vi "TestNewStructure.vi"() -> ()   [LabVIEW 2024]
uses:
  Library/Class/Renishaw-XL80_EMU/Renishaw-XL80_EMU.lvclass
panel:
  in  "Reset":bool
  out "Record":dbl
  out "GetLaserMeasurement 2":dbl
  out "Connect 2":bool
  in  "Boolean":bool
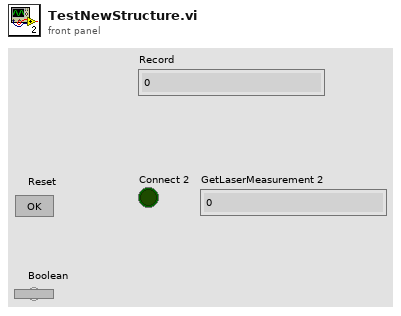
[diagram p1: front panel]
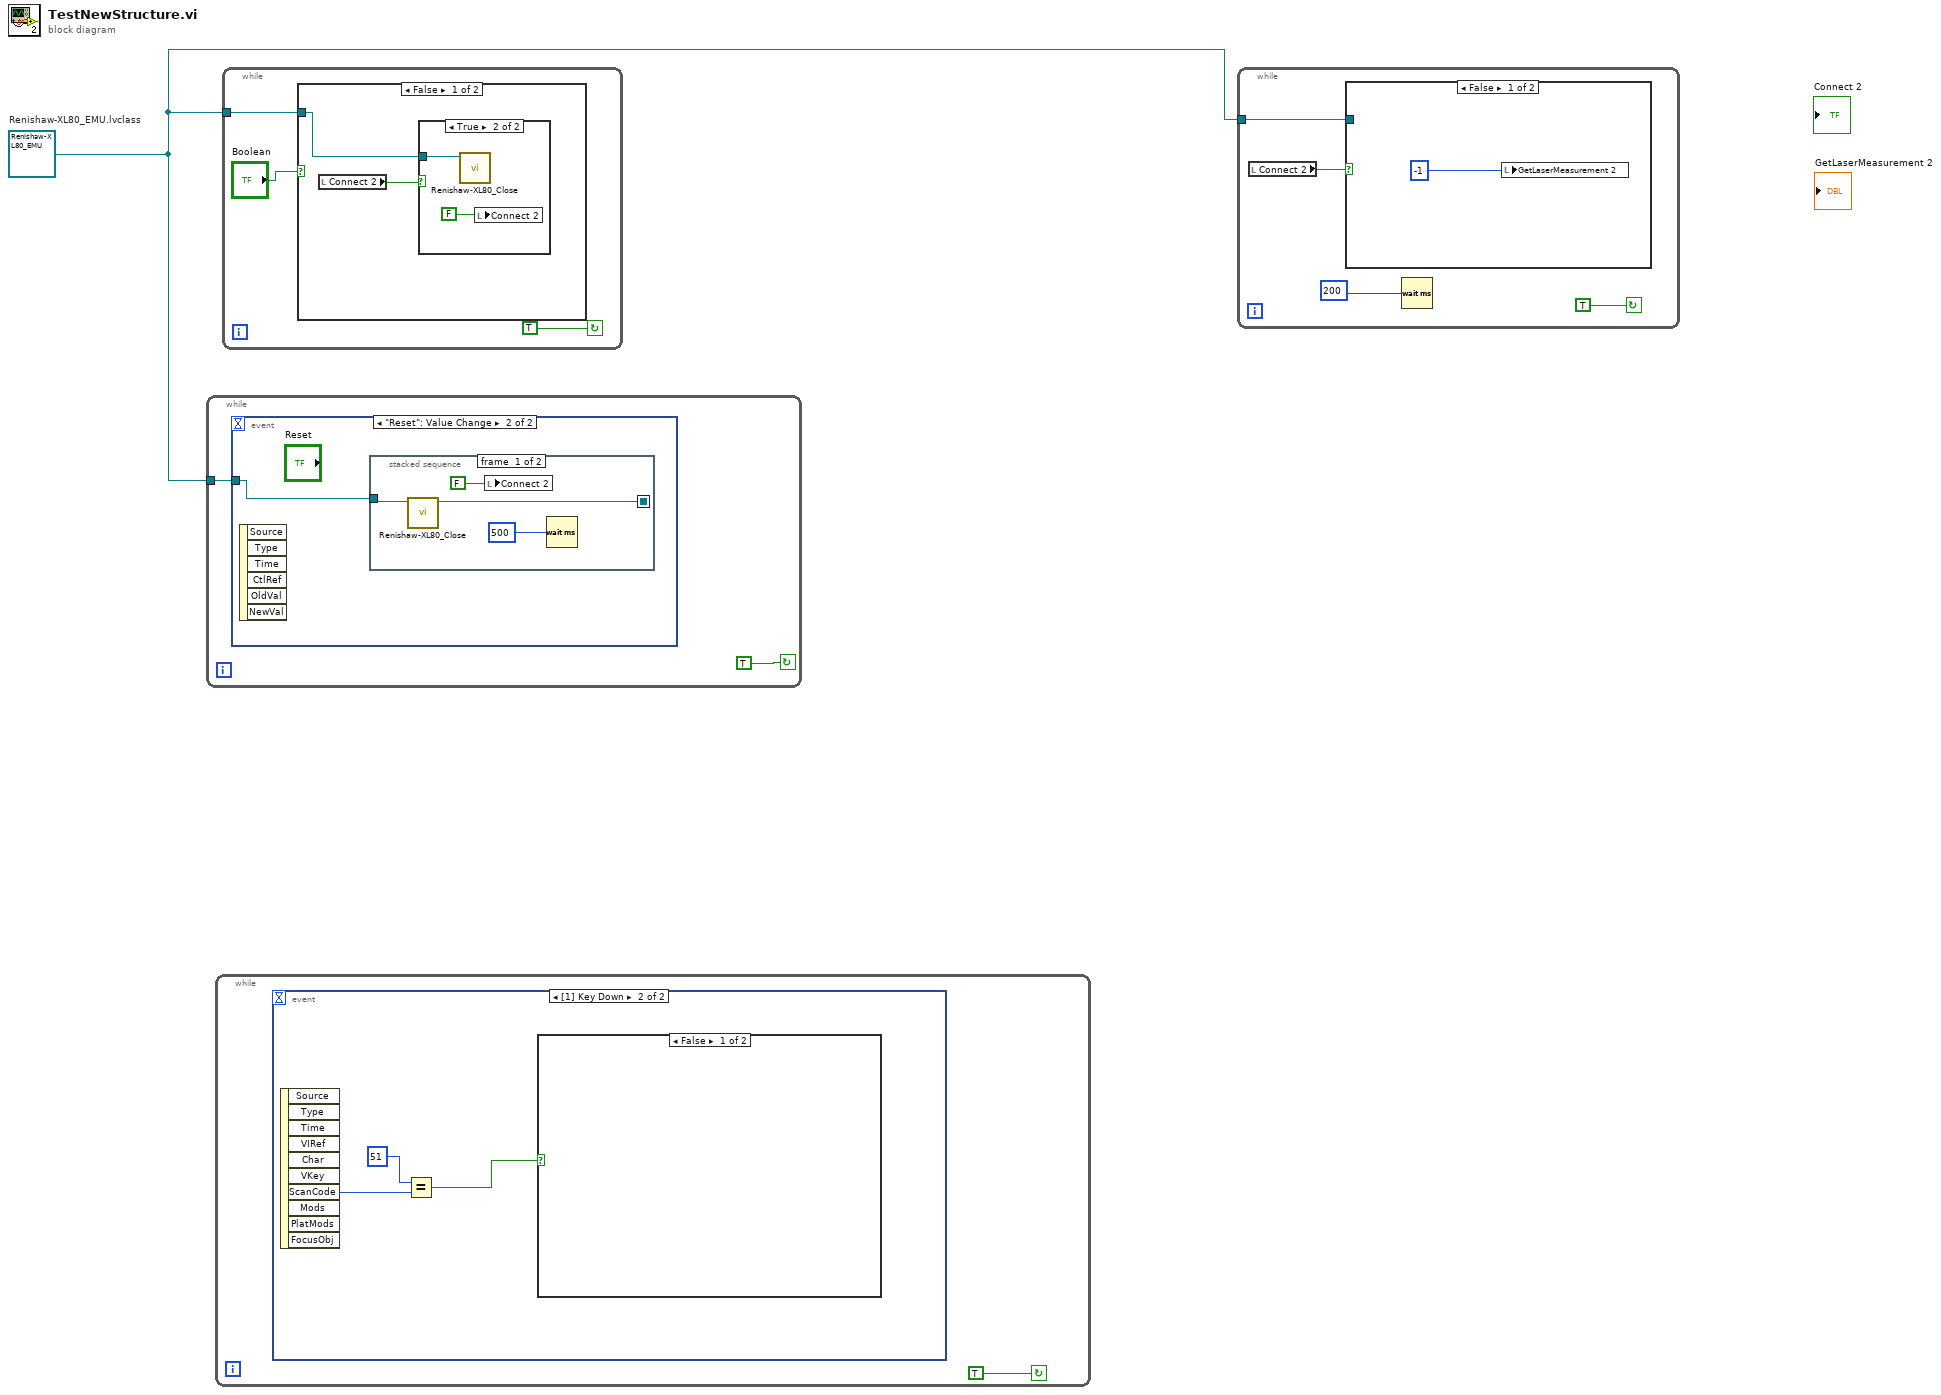
[diagram p0: block diagram]
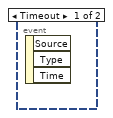
[diagram p2: hidden frame]
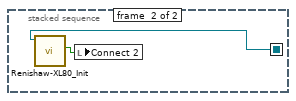
[diagram p3: hidden frame]
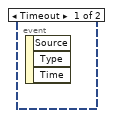
[diagram p4: hidden frame]
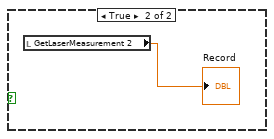
[diagram p5: hidden frame]
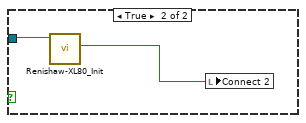
[diagram p7: hidden frame]
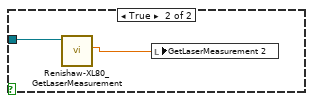
[diagram p8: hidden frame]
diagram:
  w1 = refnum<class "Renishaw-XL80_EMU.lvclass"> refnum  # Renishaw-XL80_EMU.lvclass
  n1 = while {
    tunnel: w1 -> [w3]
    stop <- TRUE continue-if-true
    n2 = event shown="[1] \"Reset\": Value Change" {
      selector: _ -> [_ _]
      dyn-events: _ -> [_ _]
      timeout: _ -> [_ _]
      tunnel: w3 -> [_ w4]
      event Timeout {
        n3 = event-data() -> ()  [unwired: 1 in, 3 out]
      }
      event "Reset": Value Change {
        n4 = event-data() -> ()  [unwired: 1 in, 6 out]
        n5 = stacked-sequence {
          seq-local: [w6 _] -> [_ w9]
          tunnel: w4 -> [w8 _]
          frame #0 {
            n6 = call-dynamic "Renishaw-XL80_Close.vi"("Renishaw-XL80_EMU in"=w8) -> ("Renishaw-XL80_EMU out"=w6:refnum<class "Renishaw-XL80_EMU.lvclass">)  [unwired: 9 in, 1 out]
            n7 = local write "Connect 2"(FALSE ("Connect 2")) -> ()
            n8 = Wait (ms)(milliseconds to wait=u32 500) -> ()  [unwired: 1 out]
          }
          frame #1 {
            n9 = call-dynamic "Renishaw-XL80_Init.vi"("Renishaw-XL80_EMU in"=w9) -> ("Connect"=w10:bool)  [unwired: 7 in, 3 out]
            n10 = local write "Connect 2"(w10) -> ()
          }
        }
      }
    }
  }
  n11 = while {
    stop <- TRUE continue-if-true
    n12 = event shown="[1] Key Down" {
      selector: _ -> [_ _]
      dyn-events: _ -> [_ _]
      timeout: _ -> [_ _]
      event Timeout {
        n13 = event-data() -> ()  [unwired: 1 in, 3 out]
      }
      event Key Down {
        n14 = event-data() -> ("ScanCode"=w13:i16)  [unwired: 1 in, 9 out]
        n15 = Equal?(x=i16 51 ("y"), y=w13) -> (x = y?=w12:bool)
        n16 = case shown="False" w12 {
          frame False {
          }
          frame True {
            n17 = local read "GetLaserMeasurement 2"() -> (→"Record":dbl)
          }
        }
      }
    }
  }
  n18 = while {
    tunnel: w1 -> [w17]
    stop <- TRUE continue-if-true
    n19 = case shown="False" "Boolean" {
      tunnel: w17 -> [w19 w23]
      frame False {
        n20 = local read "Connect 2"() -> (w20:bool)
        n21 = case shown="True" w20 {
          tunnel: w19 -> [_ w22]
          frame False {
          }
          frame True {
            n22 = call-dynamic "Renishaw-XL80_Close.vi"("Renishaw-XL80_EMU in"=w22) -> ()  [unwired: 9 in, 2 out]
            n23 = local write "Connect 2"(FALSE ("Connect")) -> ()
          }
        }
      }
      frame True {
        n24 = call-dynamic "Renishaw-XL80_Init.vi"("Renishaw-XL80_EMU in"=w23) -> ("Connect"=w24:bool)  [unwired: 7 in, 3 out]
        n25 = local write "Connect 2"(w24) -> ()
      }
    }
  }
  n26 = while {
    tunnel: w1 -> [w28]
    stop <- TRUE continue-if-true
    n27 = local read "Connect 2"() -> (w27:bool)
    n28 = case shown="False" w27 {
      tunnel: w28 -> [_ w31]
      frame False {
        n29 = local write "GetLaserMeasurement 2"(-1) -> ()
      }
      frame True {
        n30 = call-dynamic "Renishaw-XL80_GetLaserMeasurement.vi"("Renishaw-XL80_EMU in"=w31) -> ("GetLaserMeasurement"=w30:dbl)  [unwired: 7 in, 3 out]
        n31 = local write "GetLaserMeasurement 2"(w30) -> ()
      }
    }
    n32 = Wait (ms)(milliseconds to wait=u32 200) -> ()  [unwired: 1 out]
  }
